vi "id参数转换.vi"(11 "id":u16) -> (3 "table输出":string, 5 "数组资源索引":i32)   [LabVIEW 2016, in "斯坦道氨氮.lvlib"]
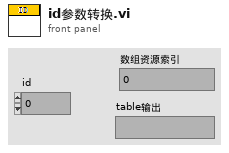
[diagram p1: front panel]
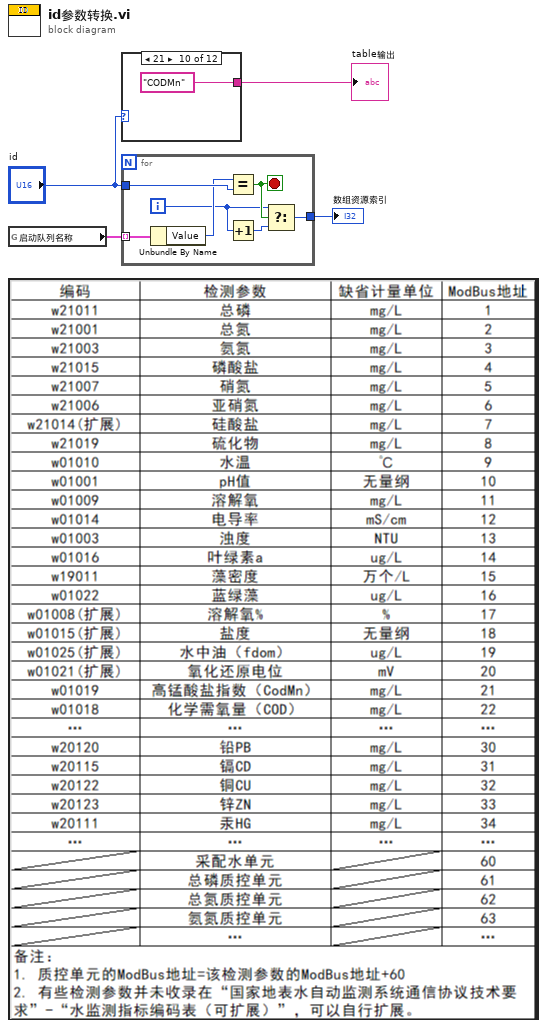
[diagram p0: block diagram]
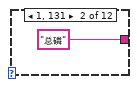
[diagram p3: hidden frame]
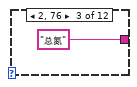
[diagram p4: hidden frame]
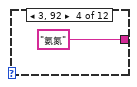
[diagram p5: hidden frame]
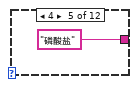
[diagram p6: hidden frame]
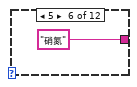
[diagram p7: hidden frame]
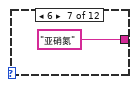
[diagram p8: hidden frame]
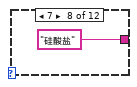
[diagram p9: hidden frame]
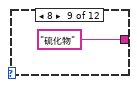
[diagram p10: hidden frame]
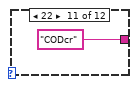
[diagram p11: hidden frame]
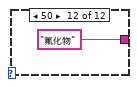
[diagram p12: hidden frame]
diagram:
  n1 = global read "model config var.vi" "启动队列名称"() -> (w3:cluster{"String":string, "Value":u16}[])
  n2 = case shown="21" "id" {
    tunnel: [_ "总磷" ("table输入") "总氮" ("table输入") "氨氮" ("table输入") "磷酸盐" ("table输入") "硝氮" ("table输入") "亚硝氮" ("table输入") "硅酸盐" ("table输入") "硫化物" ("table输入") "CODMn" ("table输入") "CODcr" ("table输入") "氟化物" ("table输入")] -> w4
    frame 0, Default {
    }
    frame 1, 131 {
    }
    frame 2, 76 {
    }
    frame 3, 92 {
    }
    frame 4 {
    }
    frame 5 {
    }
    frame 6 {
    }
    frame 7 {
    }
    frame 8 {
    }
    frame 21 {
    }
    frame 22 {
    }
    frame 50 {
    }
  }
  "table输出" <- w4
  n3 = for {
    tunnel: w3 -> [w22] mode=indexing
    tunnel: "id" -> [w21]
    tunnel: [w16] -> w1
    i -> [w17]
    stop <- w19 stop-if-true
    n4 = Unbundle By Name(w22) -> ("Value"=w20:u16)
    n5 = Equal?(x=w20, y=w21) -> (x = y?=w19:bool)
    n6 = Increment(x=w17) -> (x+1=w18:i32)
    n7 = Select(t=w17, s=w19, f=w18) -> (s? t:f=w16:i32)
  }
  "数组资源索引" <- w1
